vi "load_presets.vi"(11 "Ring in":refnum<vi>) -> ()   [LabVIEW 2011]
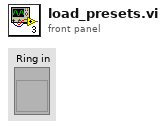
[diagram p1: front panel]
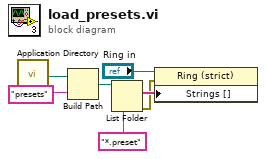
[diagram p0: block diagram]
diagram:
  n1 = call <vilib>:"Application Directory.vi"() -> ("Application Directory"=w3:path)
  n2 = Build Path(base path=w3, name or relative path="presets") -> (appended path=w5:path)
  n3 = List Folder(path=w5, pattern="*.preset") -> (filenames=w7:string[], error out=w6:errorcluster)  [unwired: 2 in, 2 out]
  n4 = property on="Property Node" class="Ring (strict)"(reference="Ring in", error in=w6, "Strings []"=w7) -> ()  [unwired: 2 out]
